vi "G#SubSubClass2_GetAttributes.vi"(0 "reference in":refnum<class "G#SubSubClass2.lvclass">, 1 "return data? (T)":bool=TRUE, 5 "error in (no error)":errorcluster) -> (14 "reference out":refnum<class "G#SubSubClass2.lvclass">, 15 "attributes ref":T4, 16 "attributes":T1, 19 "error out":errorcluster)   [LabVIEW 2017, in "G#SubSubClass2.lvclass"]
doc: "Returns a reference and if wanted the actual data values of the attributes. This method is used by the subclasses to access parent attributes."
uses:
  G#SubSubClass2.lvclass
  C:/Projects/GsharpGIT2017/Verification/TestCases/TestClasses/G#SubClass2_class/G#SubClass2.lvclass
  ObjectAttributesRef.ctl
  protected/ObjectAttributes.ctl
  G#SubClass2_class/protected/ObjectAttributes.ctl
  G#BaseClass2_class/protected/ObjectAttributes.ctl
  G#SubSubClass2.lvclass/G#SubSubClass2.ctl
  G#SubClass2_class/G#SubClass2.lvclass
  G#BaseClass2_class/G#BaseClass2.lvclass
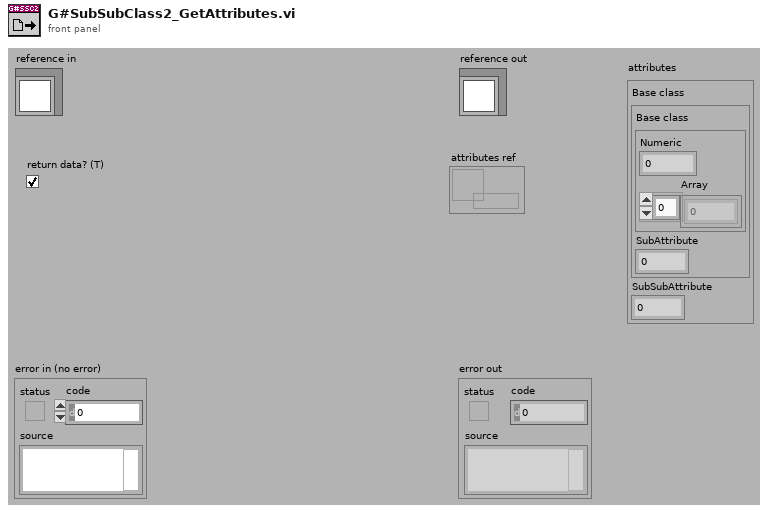
[diagram p1: front panel]
types:
  T1 = typedef "G#SubSubClass2.lvclass/ObjectAttributes.ctl" = cluster{"Base class":T2, "SubSubAttribute":dbl}
  T2 = typedef "G#SubClass2.lvclass/ObjectAttributes.ctl" = cluster{"Base class":T3, "SubAttribute":dbl}
  T3 = typedef "G#BaseClass2.lvclass/ObjectAttributes.ctl" = cluster{"Numeric":dbl, "Array":dbl[]}
  T4 = typedef "G#SubSubClass2.lvclass/ObjectAttributesRef.ctl" = refnum<data-value>
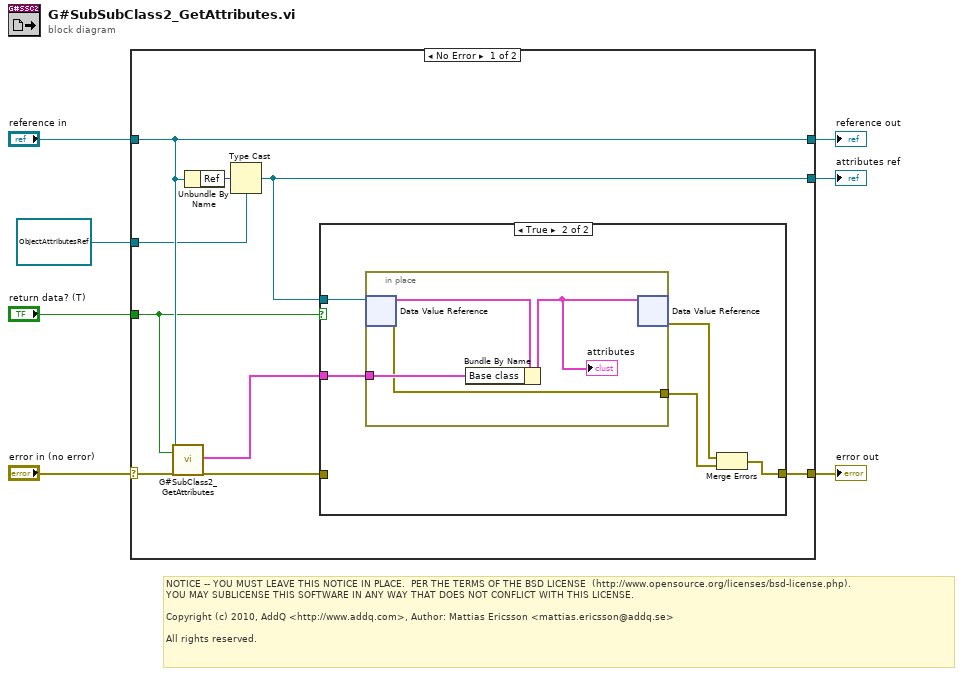
[diagram p0: block diagram]
diagram:
  # "NOTICE -- YOU MUST LEAVE THIS NOTICE IN PLACE.  PER THE TERMS OF THE BSD LICENSE  (http://www.opensource.org/licenses/bsd-license.php).\nYOU MAY SUBLICENSE THIS SOFTWARE IN ANY WAY THAT DOES NOT CONFLICT WITH THIS LICENSE.\n\nCopyright (c) 2010, AddQ <http://www.addq.com>, Author: Mattias Ericsson <mattias.ericsson@addq.se>\n\nAll rights reserved."
  n1 = case shown="No Error" "error in (no error)" {
    selector: "error in (no error)" -> [w15 w29]
    tunnel: [w16 w29] -> w6
    tunnel: [w13 w28] -> w4
    tunnel: "reference in" -> [w13 w28]
    tunnel: [w9 w27] -> w3
    tunnel: "return data? (T)" -> [w12 _]
    tunnel: T4 refnum ("attributes ref") -> [w8 w27]
    frame No Error {
      n2 = call "G#SubClass2_GetAttributes.vi"("reference in"=w13, "return data? (T)"=w12, "error in (no error)"=w15) -> ("attributes"=w11:T2, "error out"=w14:errorcluster)  [unwired: 13 in, 2 out]
      n3 = Unbundle By Name(w13) -> ("Ref"=w10:u32)
      n4 = Type Cast(type=w8, x=w10) -> (*(type *) &x=w9:T4)
      n5 = case shown="True" w12 {
        tunnel: w9 -> [_ w22]
        tunnel: w14 -> [w17 _]
        tunnel: [w17 w19] -> w16
        tunnel: w11 -> [_ w18]
        frame False {
        }
        frame True {
          n6 = in-place {
            in-place-border: [w23] -> w21
            in-place-border: w18 -> [w24]
            n7 = in-place-dvr #1(w22) -> (w26:T1, w23:errorcluster)
            n8 = Bundle By Name(cluster=w26, "Base class"=w24) -> (w25:T1)
            "attributes" <- w25
            n9 = in-place-dvr #1(w25) -> (w20:errorcluster)  [unwired: 1 out]
          }
          n10 = Merge Errors(w20, w21) -> (w19:errorcluster)
        }
      }
    }
    frame Error {
    }
  }
  "error out" <- w6
  "reference out" <- w4
  "attributes ref" <- w3
